vi "To JSON.vi"(8 "Error In":errorcluster, 10 "File Path":path, 11 "object in":refnum<class "Continuous Waveform Acq CFG.lvclass">) -> (0 "Error Out":errorcluster, 3 "object out":refnum<class "Continuous Waveform Acq CFG.lvclass">)   [LabVIEW 2023, in "PXIe-5172 Simulated.lvlib" / "Continuous Waveform Acq CFG.lvclass"]
uses:
  Continuous Waveform Acq CFG.lvclass
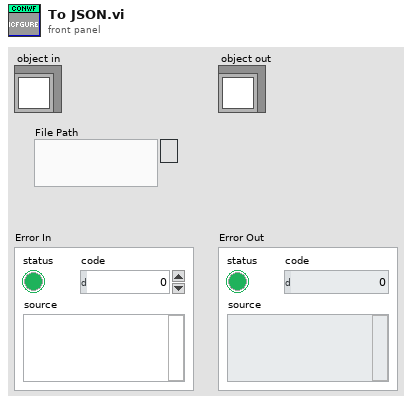
[diagram p1: front panel]
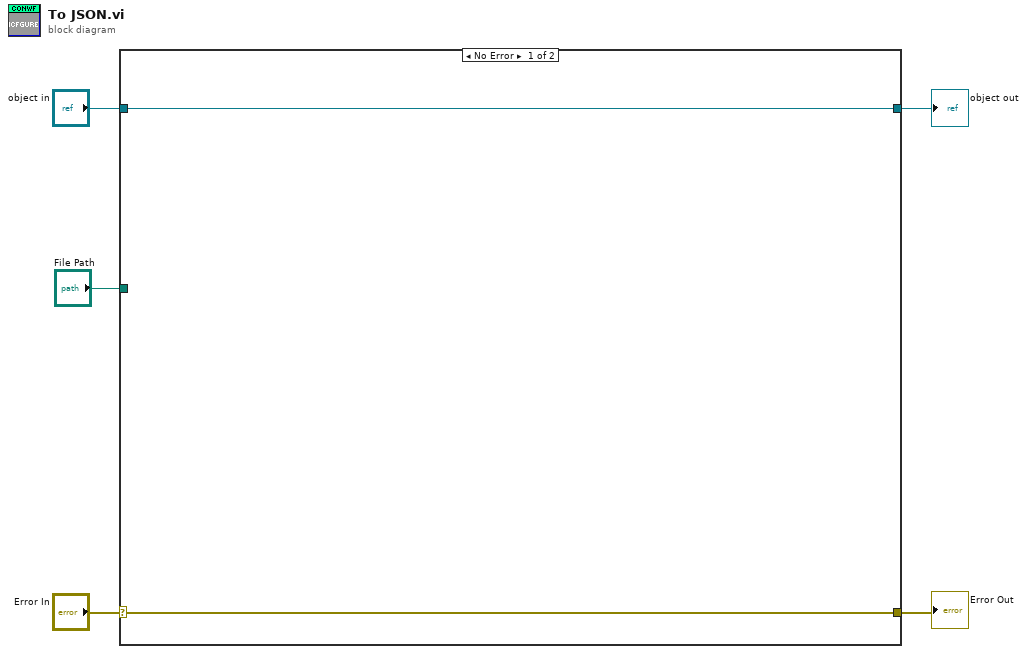
[diagram p0: block diagram]
diagram:
  n1 = case shown="No Error" "Error In" {
    selector: "Error In" -> [w6 w8]
    tunnel: [w6 w8] -> w4
    tunnel: [w7 w9] -> w2
    tunnel: "object in" -> [w7 w9]
    tunnel: "File Path" -> [_ _]
    frame No Error {
    }
    frame Error {
    }
  }
  "Error Out" <- w4
  "object out" <- w2
